vi "FG Motor Communication Sessions.vi"(7 "action":T1, 8 "error in (no error)":errorcluster, 10 "motor name":string, 11 "motor communication in":refnum<class "NI_Robotics_Motor Communication.lvclass">) -> (0 "error out":errorcluster, 1 "failed?":bool, 3 "motor communication out":refnum<class "NI_Robotics_Motor Communication.lvclass">)   [LabVIEW 2017, in "NI_Robotics_Motor Communication.lvclass"]
uses:
  <vilib>/robotics/Actuation/Motor Communication/NI_Robotics_Motor Communication.lvclass
  <vilib>/robotics/Actuation/Motor Communication/FG Motor Comm Sessions Action.ctl
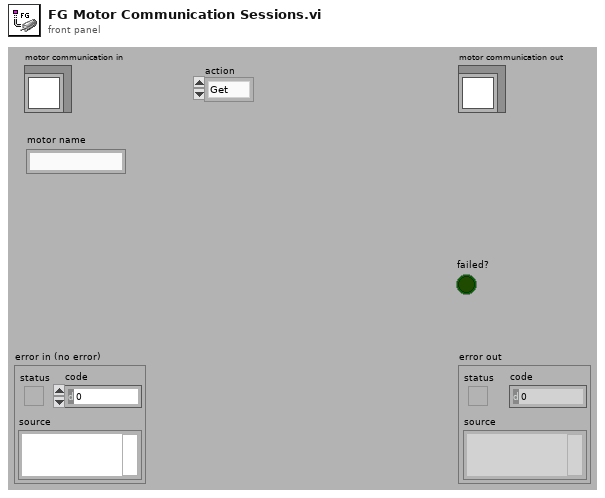
[diagram p1: front panel]
types:
  T1 = typedef "NI_Robotics_Motor Communication.lvclass/FG Motor Comm Sessions Action.ctl" = enum16{"Get", "Add", "Delete"}
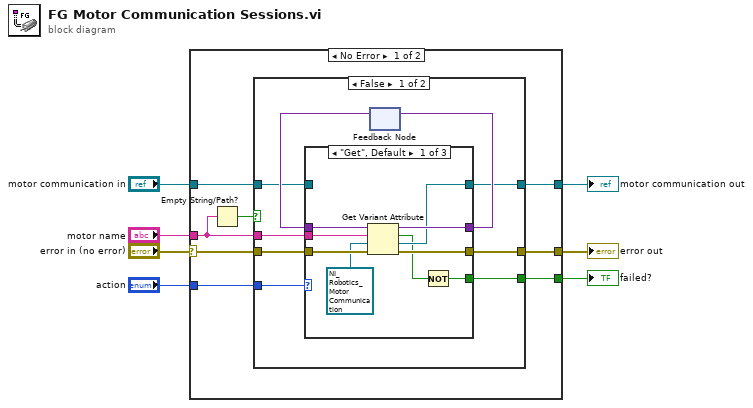
[diagram p0: block diagram]
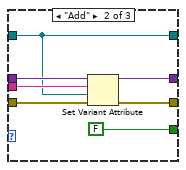
[diagram p2: hidden frame]
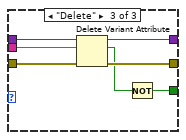
[diagram p3: hidden frame]
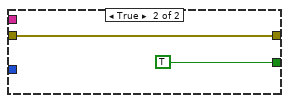
[diagram p4: hidden frame]
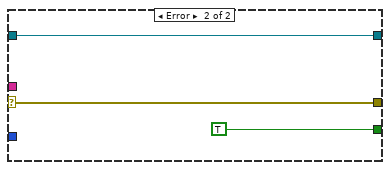
[diagram p5: hidden frame]
diagram:
  n1 = case shown="No Error" "error in (no error)" {
    selector: "error in (no error)" -> [w14 w52]
    tunnel: [w13 w52] -> w6
    tunnel: "action" -> [w15 _]
    tunnel: "motor name" -> [w9 _]
    tunnel: [w12 w51] -> w3
    tunnel: [w11 TRUE ("replaced")] -> w2
    tunnel: "motor communication in" -> [w10 w51]
    frame No Error {
      n2 = Empty String/Path?(string/path=w9) -> (empty?=w8:bool)
      n3 = case shown="False" w8 {
        tunnel: w15 -> [w24 _]
        tunnel: w14 -> [w23 w48]
        tunnel: [w20 w48] -> w13
        tunnel: [w19 _] -> w12
        tunnel: [w18 TRUE] -> w11
        tunnel: w10 -> [w17 _]
        tunnel: w9 -> [w16 _]
        frame False {
          n4 = feedback #1() -> (w21:variant)  [unwired: 1 in]
          n5 = case shown="\"Get\", Default" w24 {
            tunnel: w23 -> [w33 w37 w45]
            tunnel: w16 -> [w32 w38 w46]
            tunnel: [w31 w39 w43] -> w22
            tunnel: w21 -> [w30 w40 w47]
            tunnel: [w29 w36 w44] -> w20
            tunnel: [w28 w35 _] -> w19
            tunnel: [w26 FALSE w41] -> w18
            tunnel: w17 -> [_ w35 _]
            frame "Get", Default {
              n6 = Get Variant Attribute(Variant=w30, name=w32, default value (empty Variant)=refnum<class "NI_Robotics_Motor Communication.lvclass"> refnum ("Motor Communication.lvclass"), error in=w33) -> (duplicate Variant=w31:variant, found=w27:bool, value=w28:refnum<class "NI_Robotics_Motor Communication.lvclass">, error out=w29:errorcluster)
              n7 = Not(x=w27) -> (.not. x?=w26:bool)
            }
            frame "Add" {
              n8 = Set Variant Attribute(Variant=w40, name=w38, value=w35, error in=w37) -> (Variant out=w39:variant, error out=w36:errorcluster)  [unwired: 1 out]
            }
            frame "Delete" {
              n9 = Delete Variant Attribute(4:w45, 6:w46, 7:w47) -> (0:w44:errorcluster, 2:w42:bool, 3:w43:variant)
              n10 = Not(x=w42) -> (.not. x?=w41:bool)
            }
          }
          n11 = feedback-in #1(w22) -> ()
        }
        frame True {
        }
      }
    }
    frame Error {
    }
  }
  "error out" <- w6
  "failed?" <- w2
  "motor communication out" <- w3
